vi "Context-Search.vi"() -> ()   [LabVIEW 2020]
uses:
  <vilib>/Utility/file.llb/Read Delimited Spreadsheet (string).vi
panel:
  in  "Context Length":i32=20
  out "Context":string[](array[string])
  out "Number of Occurrences":i32
  out "Word Found in Text":bool
  in  "Selected Word":i32
  out "All Words":string[](array[string])
  out "Text to Scan":string
  in  "File to Scan":path
  in  "Search Word File":path
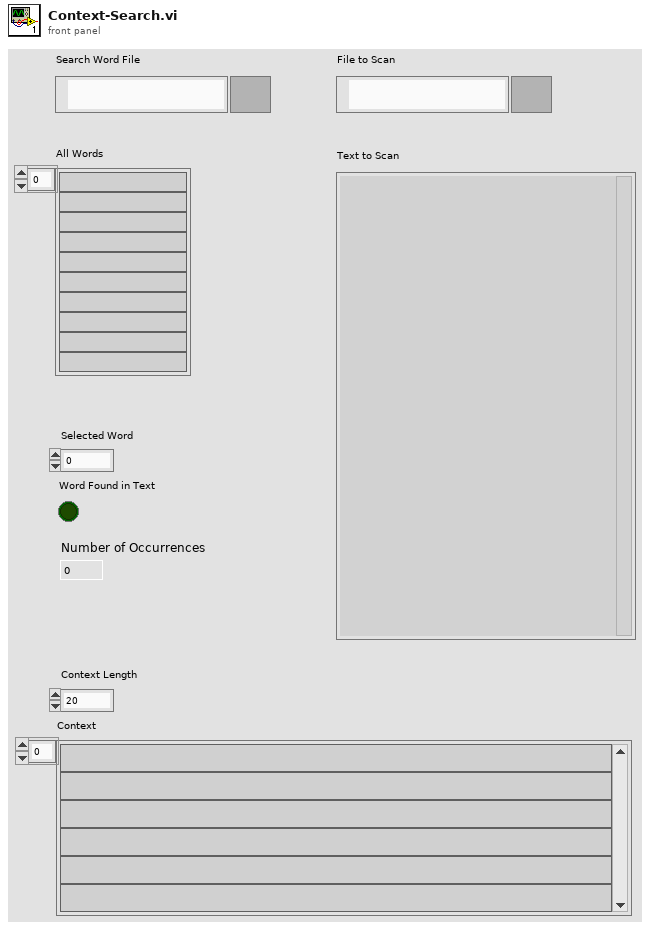
[diagram p1: front panel]
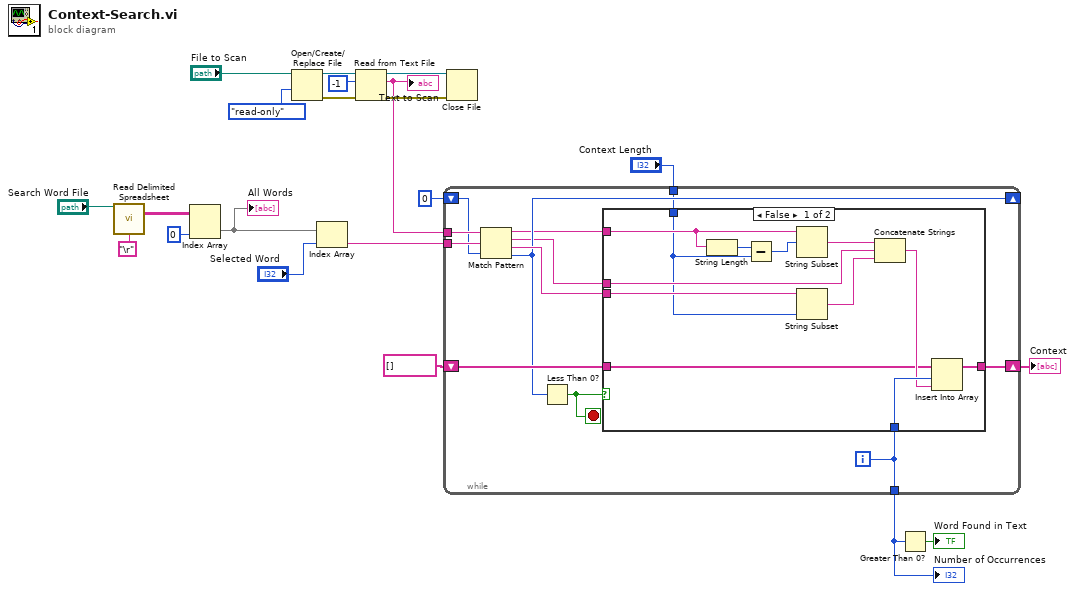
[diagram p0: block diagram]
diagram:
  n1 = call-poly <vilib>:"Read Delimited Spreadsheet.vi"("file path (dialog if empty)"="Search Word File", "delimiter (\\t)"="\r") -> ("all rows"=w13:string[][])  [unwired: 8 in, 5 out]
  n2 = Index Array(array=w13, index (col)=0 ("disabled index (col)")) -> (element=w9:string[])  [unwired: 1 in]
  "All Words" <- w9
  n3 = Open/Create/Replace File(file path (use dialog)="File to Scan", access (0:read/write)=enum16{"read/write", "read-only", "write-only"}."read-only") -> (refnum out=w21:refnum<file>, error out=w20:errorcluster)  [unwired: 4 in, 1 out]
  n4 = Index Array(array=w9, index="Selected Word") -> (element=w7:string)
  n5 = Read from Text File(file (use dialog)=w21, count=-1, error in=w20) -> (refnum out=w19:refnum<file>, text=w8:string, error out=w18:errorcluster)  [unwired: 1 in, 1 out]
  "Text to Scan" <- w8
  n6 = while {
    tunnel: w8 -> [w33]
    tunnel: w7 -> [w32]
    shift-right: [w29] -> w3
    shift-left: string[] [] -> [w30]
    shift-right: [w27] -> _
    shift-left: 0 ("dimension size") -> [w28]
    tunnel: [w26] -> w5
    tunnel: "Context Length" -> [w22]
    i -> [w26]
    stop <- w24 stop-if-true
    n7 = Match Pattern(string=w33, regular expression=w32, offset (0)=w28) -> (before substring=w25:string, match substring=w23:string, after substring=w31:string, offset past match=w27:i32)
    n8 = Less Than 0?(x=w27) -> (x < 0?=w24:bool)
    n9 = case shown="False" w24 {
      tunnel: w31 -> [w43 _]
      tunnel: w30 -> [w35 w46]
      tunnel: [w42 w46] -> w29
      tunnel: w26 -> [w41 _]
      tunnel: w25 -> [w40 _]
      tunnel: w23 -> [w38 _]
      tunnel: w22 -> [w34 _]
      frame False {
        n10 = String Length(string=w40) -> (length=w45:i32)
        n11 = Subtract(x=w45, y=w34) -> (x-y=w44:i32)
        n12 = String Subset(string=w40, offset (0)=w44) -> (substring=w39:string)  [unwired: 1 in]
        n13 = String Subset(string=w43, length (rest)=w34) -> (substring=w37:string)  [unwired: 1 in]
        n14 = Concatenate Strings(w39, w38, w37) -> (w36:string)
        n15 = Insert Into Array(array=w35, index=w41, new element=w36) -> (w42:string[])
      }
      frame True {
      }
    }
  }
  "Number of Occurrences" <- w5
  "Context" <- w3
  n16 = Close File(refnum=w19, error in=w18) -> ()  [unwired: 2 out]
  n17 = Greater Than 0?(x=w5) -> (x > 0?=→"Word Found in Text":bool)
